vi "getColor.vi"(8 "error in (no error)":errorcluster, 10 "Color":string, 11 "ShapeFactory in":refnum<class "ShapeFactory.lvclass">) -> (0 "error out":errorcluster, 2 "afColor.lvclass":refnum<class "afColor.lvclass">, 3 "ShapeFactory out":refnum<class "ShapeFactory.lvclass">)   [LabVIEW 2017, in "ShapeFactory.lvclass"]
uses:
  ShapeFactory.lvclass
  afColor Class/afColor.lvclass
  AbstractFactory Class/AbstractFactory.lvclass
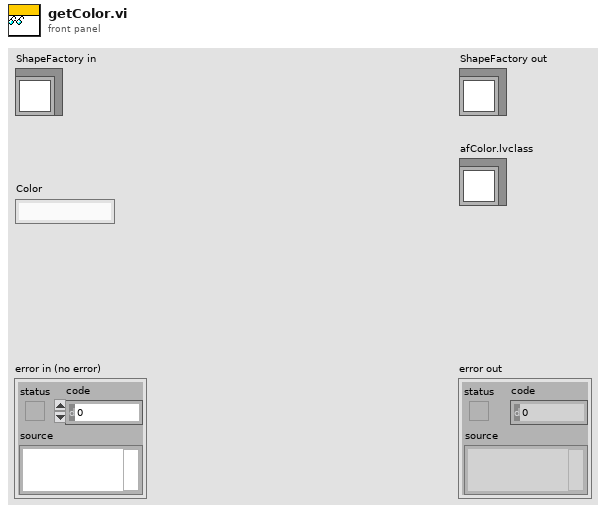
[diagram p1: front panel]
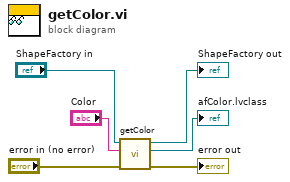
[diagram p0: block diagram]
diagram:
  n1 = call-parent "getColor.vi"("error in (no error)"="error in (no error)", "Color"="Color", "AbstractFactory in"="ShapeFactory in") -> ("error out"=→"error out":errorcluster, "afColor.lvclass"=→"afColor.lvclass":refnum<class "afColor.lvclass">, "AbstractFactory out"=→"ShapeFactory out":refnum<class "ShapeFactory.lvclass">)  [unwired: 6 in]
